vi "libssh2_channel_direct_tcpip.vi"(8 "error in (no error)":errorcluster, 9 "port":i32, 10 "host":string, 11 "session":T2) -> (0 "error out":errorcluster, 3 "channel":T1)   [LabVIEW 2013, in "libssh2.lvlib"]
doc: "Create a channel to tunnel a TCP connection from local port 22 to a target host through an SSH session. Communication to the SSH server remains encrypted. Communication from the SSH server to the target host happens in clear text."
uses:
  libssh2.lvlib
  Session Refnum.ctl
  Channel Refnum.ctl
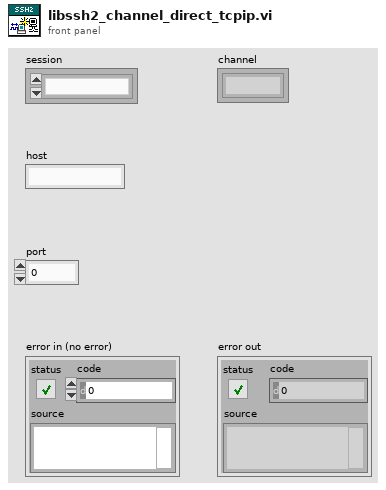
[diagram p1: front panel]
types:
  T1 = typedef "libssh2.lvlib/Channel Refnum.ctl" = refnum<k1>
  T2 = typedef "libssh2.lvlib/Session Refnum.ctl" = refnum<k1>
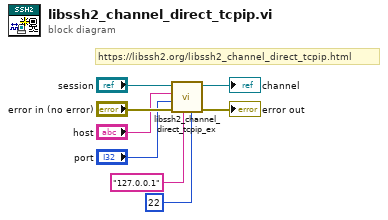
[diagram p0: block diagram]
diagram:
  # "https://libssh2.org/libssh2_channel_direct_tcpip.html"
  n1 = call "libssh2_channel_direct_tcpip_ex.vi"("sport"=22, "shost"="127.0.0.1", "error in (no error)"="error in (no error)", "port"="port", "host"="host", "session"="session") -> ("error out"=→"error out":errorcluster, "channel"=→"channel":T1)  [unwired: 4 in]
